vi "Convert String Array to Commalist String.vi"(1 "Add space between elements? (TRUE)":bool=TRUE, 2 "String Array":string[](array[string])) -> (0 "Commalist string":string)   [LabVIEW 2023, in "Error Manager.lvlib" / "Settings.lvclass"]
uses:
  Settings.lvclass
panel:
  # "Output\nOutputs of the VI"
  # "Input\nInputs to the VI"
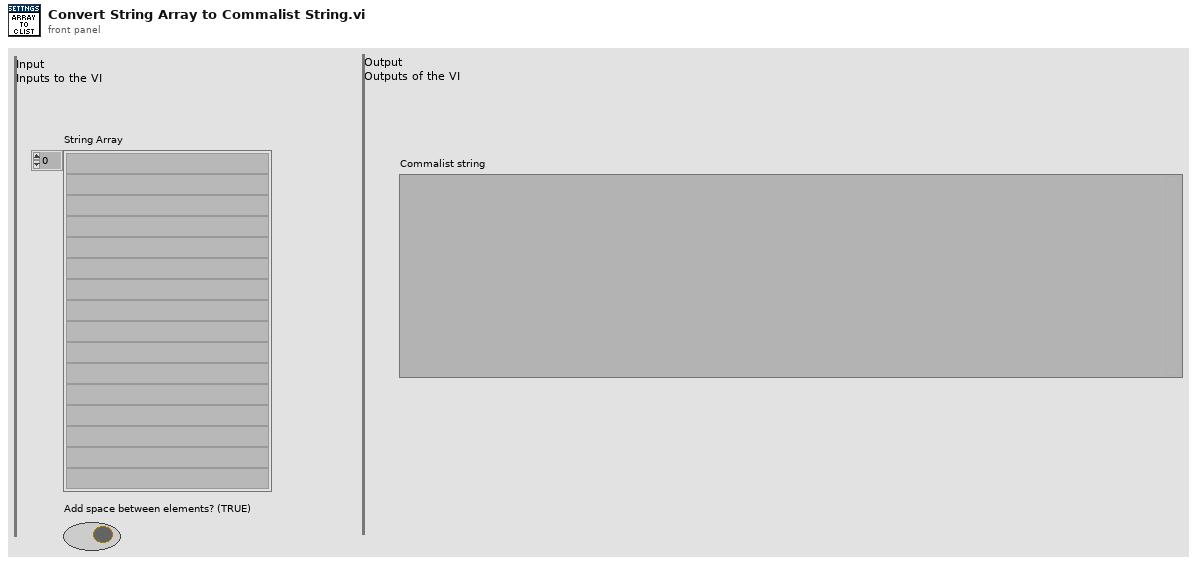
[diagram p1: front panel]
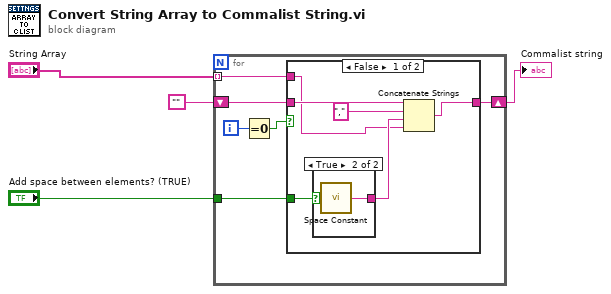
[diagram p0: block diagram]
diagram:
  n1 = for {
    tunnel: "String Array" -> [w8] mode=indexing
    shift-right: [w7] -> w3
    shift-left: "" -> [w6]
    tunnel: "Add space between elements? (TRUE)" -> [w5]
    i -> [w10]
    n2 = Equal To 0?(x=w10) -> (x = 0?=w9:bool)
    n3 = case shown="False" w9 {
      tunnel: w8 -> [w13 w18]
      tunnel: [w12 w18] -> w7
      tunnel: w6 -> [w16 _]
      tunnel: w5 -> [w11 _]
      frame False {
        n4 = case shown="True" w11 {
          tunnel: [_ w17] -> w14
          frame False {
          }
          frame True {
            n5 = call <vilib>:"Space Constant.vi"() -> ("String"=w17:string)
          }
        }
        n6 = Concatenate Strings(w16, "," ("string"), w14, w13) -> (w12:string)
      }
      frame True {
      }
    }
  }
  "Commalist string" <- w3
